vi "Mux1.vi"(1 "B":bool, 2 "A":bool, 3 "s0":bool) -> (0 "z":bool)   [LabVIEW 2012]
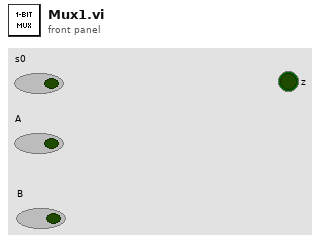
[diagram p1: front panel]
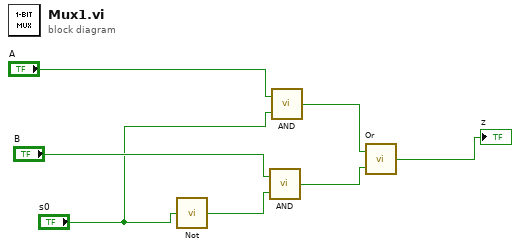
[diagram p0: block diagram]
diagram:
  n1 = call "Not.vi"("In"="s0") -> ("Out"=w7:bool)
  n2 = call "AND.vi"("b"=w7, "a"="B") -> ("x"=w2:bool)
  n3 = call "AND.vi"("b"="s0", "a"="A") -> ("x"=w3:bool)
  n4 = call "Or.vi"("b"=w2, "a"=w3) -> ("x"=→"z":bool)
